vi "Hi_Tec_Control.vi"(0 "Carrier 1 Voltage":dbl(knob) min=0.0 max=5.0 scale=0.0..5.0 scale format="%.1f", 1 "Carrier 2 Voltage":dbl(knob) min=0.0 max=5.0 scale=0.0..5.0 scale format="%.1f", 2 "Trace Voltage":dbl(knob) min=0.0 max=5.0 scale=0.0..5.0 scale format="%.1f", 3 "Trace_2 Voltage":dbl(knob) min=0.0 max=5.0 scale=0.0..5.0 scale format="%.1f", 4 "Client Name":string) -> (5 "Scan Comments":string)   [LabVIEW 2015]
uses:
  ADAM Client/Sub VIs/Channel_State_Control.ctl
  Anemometry/Anemometry Sub Vis/Controls/In_Range.ctl
  ADAM Client/Sub VIs/ADAM Controls/Update_scan_value.ctl
panel:
  out "Second stage":dbl[][](graph)
  out "First stage":dbl[][](graph)
  out "Increasing trace":bool
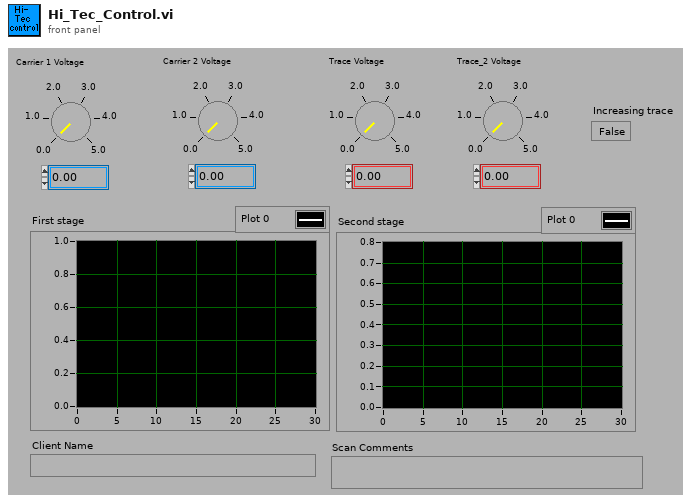
[diagram p1: front panel]
types:
  T1 = typedef "Channel_State_Control.ctl" = enum16{"Channel Name", "Channel Name Starts with", "Main Address"}
  T2 = typedef "In_Range.ctl" = enum16{"%", "±", "% & ±"}
  T3 = typedef "Update_scan_value.ctl" = cluster{"Channel Name":string, "New Value":dbl}
  T4 = enum16{"Append to Global", "Read Global then Clear"}
  T5 = typedef "Ch_description_ADAM.ctl" = cluster{"Ch Name":string, "Type":T6, "Function":T7, "Ch State":T8, "Calibration type":T9, "A":dbl, "B":dbl, "C":dbl, "D":dbl, "Comments":string, "Address":T10, "String":string, "Duty":u16}
  T6 = typedef "Module_type_ADAM.ctl" = string
  T7 = typedef "Function_ADAM.ctl" = enum16{"Analogue Input", "Digital Input", "Event counter", "Event rate", "Analogue Output", "Digital Output", "Relay Output"}
  T8 = typedef "Channel_State.ctl" = enum16{"On", "Off", "Always On", "Always Off"}
  T9 = typedef "Calib_type_ADAM.ctl" = enum16{"Raw", "Bx + A", "Cx^2 + Bx + A", "Dx^3 + Cx^2 + Bx + A", "In Band", "Hi-Tec Q", "Hi-Tec M_dot", "Text"}
  T10 = typedef "Address.ctl" = cluster{"Main":i32, "Ch.":i32, "Sub":i32, "Port Name":string}
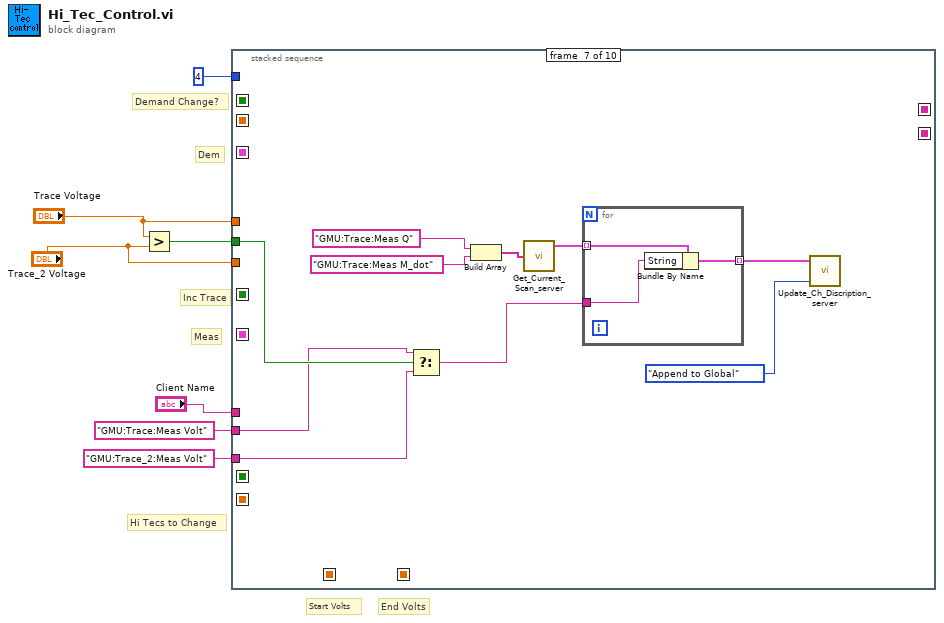
[diagram p0: block diagram]
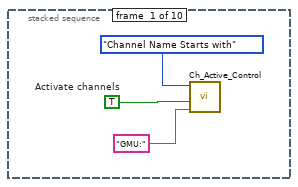
[diagram p2: hidden frame]
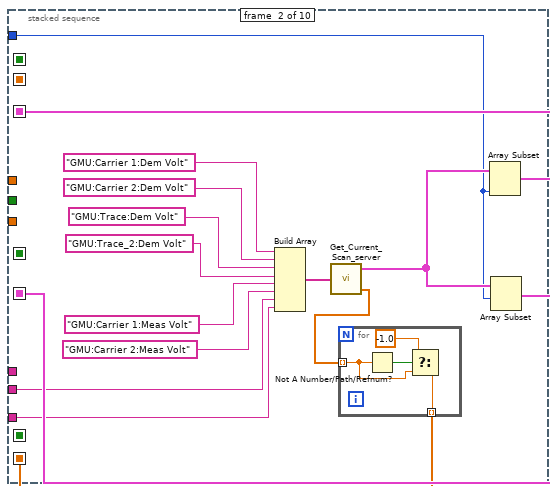
[diagram p3: hidden frame]
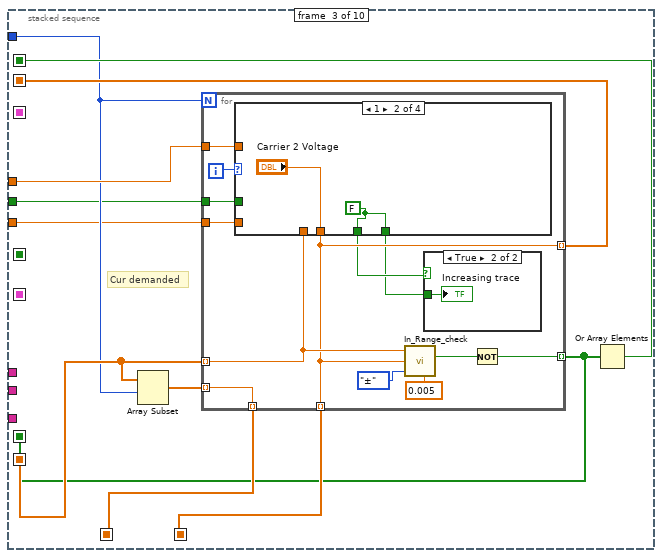
[diagram p4: hidden frame]
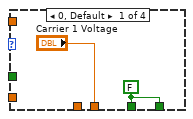
[diagram p6: hidden frame]
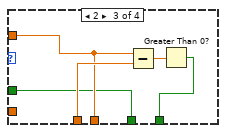
[diagram p7: hidden frame]
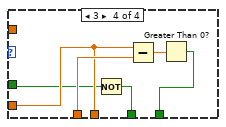
[diagram p8: hidden frame]
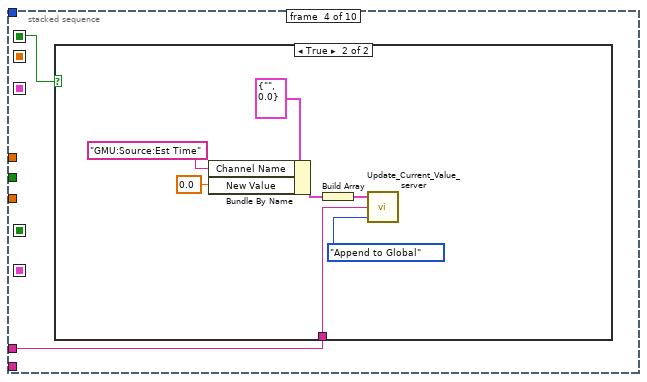
[diagram p9: hidden frame]
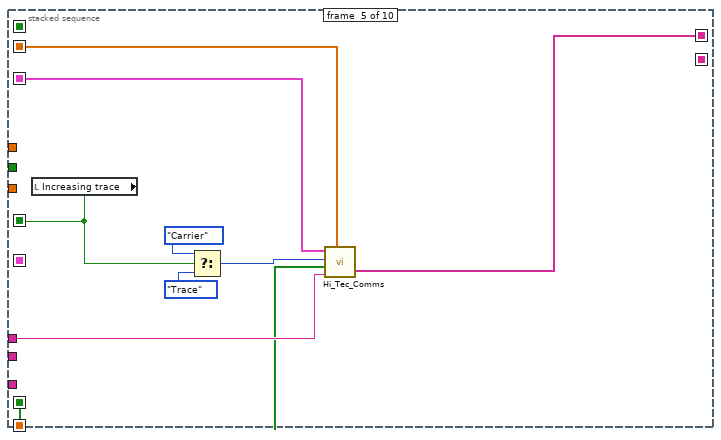
[diagram p11: hidden frame]
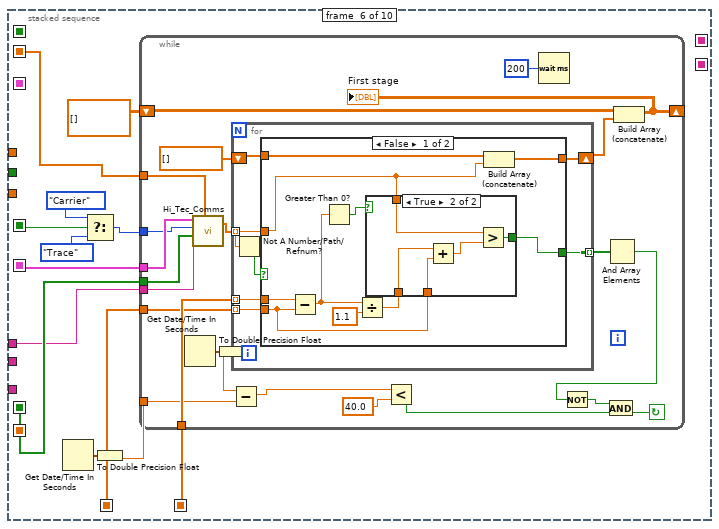
[diagram p12: hidden frame]
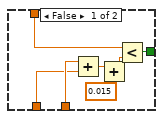
[diagram p13: hidden frame]
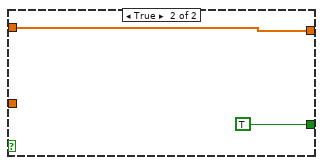
[diagram p14: hidden frame]
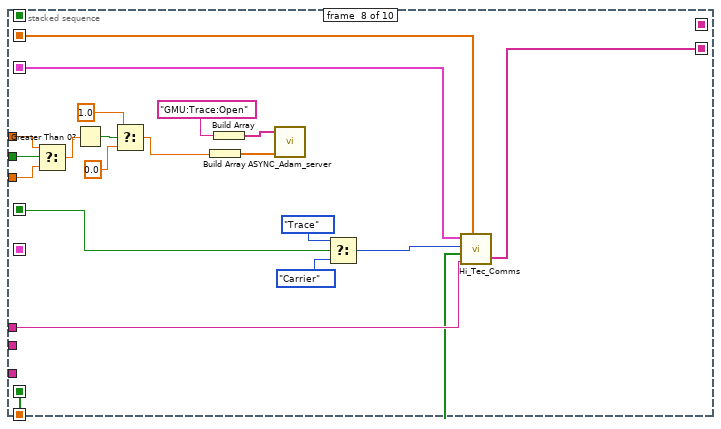
[diagram p15: hidden frame]
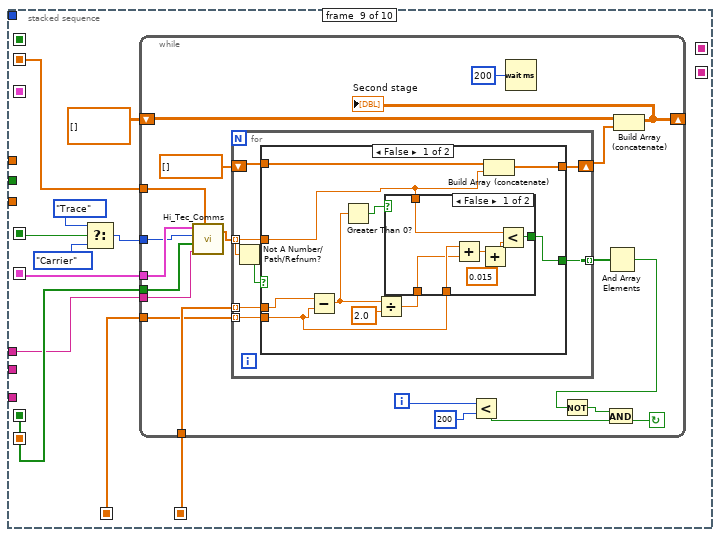
[diagram p16: hidden frame]
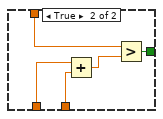
[diagram p17: hidden frame]
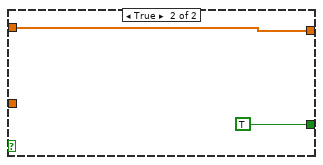
[diagram p18: hidden frame]
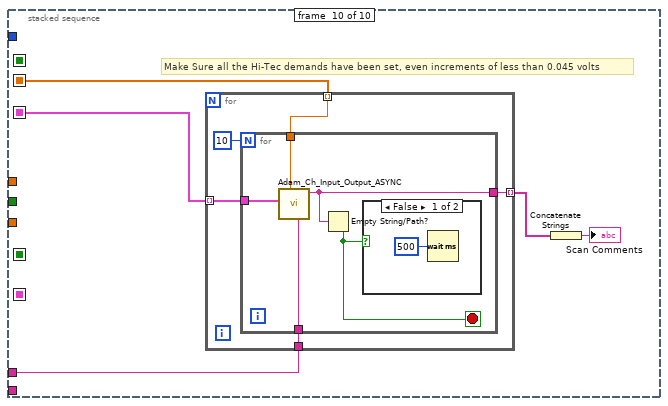
[diagram p19: hidden frame]
diagram:
  # "Dem"
  # "Demand Change?"
  # "End Volts"
  # "Start Volts"
  # "Inc Trace"
  # "Meas"
  # "Hi Tecs to Change"
  n1 = Greater?(x="Trace Voltage", y="Trace_2 Voltage") -> (0:w4:bool)
  n2 = stacked-sequence {
    seq-local: [_ w21 _ _ _ _ _ _ _ _] -> [_ _ _ _ w81 _ _ w174 _ w253]
    seq-local: [_ w16 _ _ _ _ _ _ _ _] -> [_ _ w38 _ _ _ _ _ _ _]
    seq-local: [_ _ w36 _ _ _ _ _ _ _] -> [_ _ _ _ w80 w100 _ w173 w198 _]
    seq-local: [_ w20 _ _ _ _ _ _ _ _] -> [_ _ _ _ _ w96 _ _ w194 _]
    seq-local: [_ _ _ _ w87 _ _ _ _ _] -> [_ _ _ _ _ w97 _ w187 w195 _]
    seq-local: [_ _ w40 _ _ _ _ _ _ _] -> [_ _ _ _ _ w93 _ _ w191 _]
    seq-local: [_ _ w39 _ _ _ _ _ _ _] -> [_ _ _ _ _ w94 _ _ w192 _]
    seq-local: [_ _ w35 _ _ _ _ _ _ _] -> [_ _ _ w70 _ _ _ _ _ _]
    seq-local: [_ _ w33 _ _ _ _ _ _ _] -> [_ _ _ _ w82 w88 _ w175 w188 w252]
    seq-local: [_ _ _ _ w79 _ _ _ _ _] -> [_ _ _ _ _ _ _ _ _ _]
    seq-local: [_ _ _ _ _ _ _ w172 _ _] -> [_ _ _ _ _ _ _ _ _ _]
    tunnel: "Client Name" -> [_ _ _ w71 w83 w90 _ w183 w189 w254]
    tunnel: "Trace Voltage" -> [_ _ w34 _ _ _ _ w170 _ _]
    tunnel: 4 ("Array Length") -> [_ w13 w32 _ _ _ _ _ _ _]
    tunnel: w4 -> [_ _ w31 _ _ _ w160 w171 _ _]
    tunnel: "Trace_2 Voltage" -> [_ _ w30 _ _ _ _ w168 _ _]
    tunnel: "GMU:Trace:Meas Volt" -> [_ w12 _ _ _ _ w159 _ _ _]
    tunnel: "GMU:Trace_2:Meas Volt" -> [_ w11 _ _ _ _ w158 _ _ _]
    frame #0 {
      w8 = TRUE  # Activate channels
      n3 = call "Ch_Active_Control.vi"("Match"="GMU:", "Activate Channels?"=w8, "Control on"=Channel_State_Control."Channel Name Starts with") -> ()  [unwired: 1 in, 2 out]
    }
    frame #1 {
      n4 = Build Array("GMU:Carrier 1:Dem Volt", "GMU:Carrier 2:Dem Volt", "GMU:Trace:Dem Volt", "GMU:Trace_2:Dem Volt", "GMU:Carrier 1:Meas Volt", "GMU:Carrier 2:Meas Volt", w12, w11) -> (w25:string[])
      n5 = call "Get_Current_Scan_server.vi"("Desired Channels"=w25) -> ("Ch Description Array"=w19:T5[], "Numerical Values"=w17:dbl[])  [unwired: 1 out]
      n6 = for {
        tunnel: w17 -> [w28] mode=indexing
        tunnel: [w27] -> w16 mode=indexing
        n7 = Not A Number/Path/Refnum?(number/path/refnum=w28) -> (NaN/Path/Refnum?=w29:bool)
        n8 = Select(t=-1.0, s=w29, f=w28) -> (s? t:f=w27:dbl)
      }
      n9 = Array Subset(array=w19, length=w13) -> (w21:T5[])  [unwired: 1 in]
      n10 = Array Subset(array=w19, index=w13) -> (w20:T5[])  [unwired: 1 in]
    }
    frame #2 {
      # "Cur demanded"
      n11 = Array Subset(array=w38, index=w32) -> (w37:dbl[])  [unwired: 1 in]
      n12 = for {
        N: w32 -> [_]
        tunnel: w38 -> [w48] mode=indexing
        tunnel: [w51] -> w40 mode=indexing
        tunnel: [w45] -> w39 mode=indexing
        tunnel: [w52] -> w36 mode=indexing
        tunnel: w37 -> [w51] mode=indexing
        tunnel: w34 -> [w46]
        tunnel: [w45] -> w33 mode=indexing
        tunnel: w31 -> [w43]
        tunnel: w30 -> [w41]
        i -> [w53]
        n13 = case shown="1" w53 {
          tunnel: ["Carrier 1 Voltage" "Carrier 2 Voltage" w61 w66] -> w45
          tunnel: w48 -> [_ _ w63 w69]
          tunnel: w46 -> [_ _ w61 _]
          tunnel: [w55 w57 w60 w64] -> w44
          tunnel: w43 -> [_ _ w60 w65]
          tunnel: [w55 w57 w59 w67] -> w42
          tunnel: w41 -> [_ _ _ w66]
          frame 0, Default {
            w55 = FALSE
          }
          frame 1 {
            w57 = FALSE
          }
          frame 2 {
            n14 = Subtract(x=w61, y=w63) -> (x-y=w62:dbl)
            n15 = Greater Than 0?(x=w62) -> (x > 0?=w59:bool)
          }
          frame 3 {
            n16 = Not(x=w65) -> (.not. x?=w64:bool)
            n17 = Subtract(x=w66, y=w69) -> (x-y=w68:dbl)
            n18 = Greater Than 0?(x=w68) -> (x > 0?=w67:bool)
          }
        }
        n19 = call "In_Range_check.vi"("±"=0.005 ("%"), "Mode"=In_Range."±", "Value"=w45, "Setpoint"=w48) -> ("In Range"=w47:bool)  [unwired: 1 in, 2 out]
        n20 = case shown="True" w44 {
          tunnel: w42 -> [_ w54]
          frame False {
          }
          frame True {
            "Increasing trace" <- w54
          }
        }
        n21 = Not(x=w47) -> (.not. x?=w52:bool)
      }
      n22 = Or Array Elements(Boolean array=w36) -> (logical OR=w35:bool)
    }
    frame #3 {
      n23 = case shown="True" w70 {
        tunnel: w71 -> [_ w78]
        frame False {
        }
        frame True {
          n24 = Bundle By Name(cluster=T3 {"Channel Name"="", "New Value"=0.0} ("Update Scan Value Cluster"), "Channel Name"="GMU:Source:Est Time", "New Value"=0.0 ("Bundle Element")) -> (w73:T3)
          n25 = Build Array(w73) -> (w72:T3[])
          n26 = call "Update_Current_Value_server.vi"("Mode"=T4."Append to Global", "Client HD name"=w78, "Update array in"=w72) -> ()  [unwired: 1 out]
        }
      }
    }
    frame #4 {
      n27 = local read "Increasing trace"() -> (w87:bool)
      n28 = Select(t=enum16{"Carrier", "Trace"}."Carrier" ("Type"), s=w87, f=enum16{"Carrier", "Trace"}."Trace" ("Type")) -> (s? t:f=w84:enum16{"Carrier", "Trace"})
      n29 = call "Hi_Tec_Comms.vi"("Ch Description Array"=w81, "Type"=w84, "Hi Tec's To Change"=w80, "Client Name"=w83, "Dem Volts"=w82) -> ("Scan comments"=w79:string[])  [unwired: 1 out]
    }
    frame #5 {
      n30 = Get Date/Time In Seconds() -> (seconds since 1Jan1904=w89:timestamp)
      n31 = Select(t=enum16{"Carrier", "Trace"}."Carrier" ("Type"), s=w97, f=enum16{"Carrier", "Trace"}."Trace" ("Type")) -> (s? t:f=w95:enum16{"Carrier", "Trace"})
      n32 = To Double Precision Float(number=w89) -> (double precision float=w91:dbl)
      n33 = while {
        tunnel: w90 -> [w104]
        tunnel: w91 -> [w107]
        shift-left: dbl[][] [] -> [w113]
        shift-right: [w112] -> _
        tunnel: w93 -> [w120]
        tunnel: w94 -> [w121]
        tunnel: w95 -> [w122]
        tunnel: w96 -> [w123]
        tunnel: w100 -> [w114]
        tunnel: w88 -> [w101]
        stop <- w109 continue-if-true
        n34 = Get Date/Time In Seconds() -> (seconds since 1Jan1904=w103:timestamp)
        n35 = call "Hi_Tec_Comms.vi"("Ch Description Array"=w123, "Type"=w122, "Hi Tec's To Change"=w114, "Client Name"=w104, "Dem Volts"=w101) -> ("Outputs"=w119:dbl[])  [unwired: 1 out]
        n36 = To Double Precision Float(number=w103) -> (double precision float=w108:dbl)
        n37 = Subtract(x=w108, y=w107) -> (x-y=w106:dbl)
        n38 = for {
          tunnel: w121 -> [w130] mode=indexing
          tunnel: w120 -> [w129] mode=indexing
          tunnel: w119 -> [w125] mode=indexing
          tunnel: [w128] -> w118 mode=indexing
          shift-right: [w126] -> w115
          shift-left: dbl[] [] -> [w127]
          n39 = Not A Number/Path/Refnum?(number/path/refnum=w125) -> (NaN/Path/Refnum?=w124:bool)
          n40 = case shown="False" w124 {
            tunnel: w130 -> [w137 _]
            tunnel: w129 -> [w133 _]
            tunnel: w125 -> [w132 _]
            tunnel: [w131 TRUE] -> w128
            tunnel: w127 -> [w136 w153]
            tunnel: [w135 w153] -> w126
            frame False {
              n41 = Subtract(x=w137, y=w133) -> (x-y=w139:dbl)
              n42 = Greater Than 0?(x=w139) -> (x > 0?=w138:bool)
              n43 = Divide(x=w139, y=1.1) -> (x/y=w134:dbl)
              n44 = case shown="True" w138 {
                tunnel: w134 -> [w146 w152]
                tunnel: w133 -> [w147 w151]
                tunnel: w132 -> [w145 w149]
                tunnel: [w144 w148] -> w131
                frame False {
                  n45 = Add(x=w147, y=w146) -> (x+y=w143:dbl)
                  n46 = Add(x=w143, y=0.015 ("x")) -> (x+y=w142:dbl)
                  n47 = Less?(x=w145, y=w142) -> (x < y?=w144:bool)
                }
                frame True {
                  n48 = Add(x=w152, y=w151) -> (x+y=w150:dbl)
                  n49 = Greater?(x=w149, y=w150) -> (0:w148:bool)
                }
              }
              n50 = Build Array (concatenate)(w136, w132) -> (w135:dbl[])
            }
            frame True {
            }
          }
        }
        n51 = Less?(x=w106, y=40.0) -> (x < y?=w111:bool)
        n52 = Wait (ms)(milliseconds to wait=u32 200) -> ()  [unwired: 1 out]
        n53 = And Array Elements(Boolean array=w118) -> (logical AND=w117:bool)
        n54 = Not(x=w117) -> (.not. x?=w110:bool)
        n55 = And(x=w110, y=w111) -> (x .and. y?=w109:bool)
        n56 = Build Array (concatenate)(w113, w115) -> (w112:dbl[][])
        "First stage" <- w112
      }
    }
    frame #6 {
      n57 = Select(t=w159, s=w160, f=w158) -> (s? t:f=w157:string)
      n58 = Build Array("GMU:Trace:Meas Q", "GMU:Trace:Meas M_dot") -> (w162:string[])
      n59 = call "Get_Current_Scan_server.vi"("Desired Channels"=w162) -> ("Ch Description Array"=w161:T5[])  [unwired: 2 out]
      n60 = for {
        tunnel: w161 -> [w167] mode=indexing
        tunnel: w157 -> [w166]
        tunnel: [w165] -> w156 mode=indexing
        n61 = Bundle By Name(cluster=w167, "String"=w166) -> (w165:T5)
      }
      n62 = call "Update_Ch_Discription_server.vi"("Mode"=T4."Append to Global", "Channels to update In"=w156) -> ()  [unwired: 1 in, 1 out]
    }
    frame #7 {
      n63 = Select(t=w170, s=w171, f=w168) -> (s? t:f=w169:dbl)
      n64 = Greater Than 0?(x=w169) -> (x > 0?=w182:bool)
      n65 = Select(t=1.0, s=w182, f=0.0) -> (s? t:f=w179:dbl)
      n66 = Build Array(w179) -> (w176:dbl[])
      n67 = Build Array("GMU:Trace:Open") -> (w177:string[])
      n68 = call "ASYNC_Adam_server.vi"("Values"=w176, "Channel Names"=w177) -> ()  [unwired: 2 in, 2 out]
      n69 = Select(t=enum16{"Carrier", "Trace"}."Trace" ("Type"), s=w187, f=enum16{"Carrier", "Trace"}."Carrier" ("Type")) -> (s? t:f=w184:enum16{"Carrier", "Trace"})
      n70 = call "Hi_Tec_Comms.vi"("Ch Description Array"=w174, "Type"=w184, "Hi Tec's To Change"=w173, "Client Name"=w183, "Dem Volts"=w175) -> ("Scan comments"=w172:string[])  [unwired: 1 out]
    }
    frame #8 {
      n71 = Select(t=enum16{"Carrier", "Trace"}."Trace" ("Type"), s=w195, f=enum16{"Carrier", "Trace"}."Carrier" ("Type")) -> (s? t:f=w193:enum16{"Carrier", "Trace"})
      n72 = while {
        tunnel: w189 -> [w201]
        shift-left: dbl[][] [] -> [w208]
        shift-right: [w202] -> _
        tunnel: w191 -> [w215]
        tunnel: w192 -> [w216]
        tunnel: w193 -> [w217]
        tunnel: w194 -> [w218]
        tunnel: w198 -> [w209]
        tunnel: w188 -> [w199]
        i -> [w204]
        stop <- w203 continue-if-true
        n73 = call "Hi_Tec_Comms.vi"("Ch Description Array"=w218, "Type"=w217, "Hi Tec's To Change"=w209, "Client Name"=w201, "Dem Volts"=w199) -> ("Outputs"=w214:dbl[])  [unwired: 1 out]
        n74 = for {
          tunnel: w216 -> [w225] mode=indexing
          tunnel: w215 -> [w224] mode=indexing
          tunnel: w214 -> [w220] mode=indexing
          tunnel: [w223] -> w213 mode=indexing
          shift-right: [w221] -> w210
          shift-left: dbl[] [] -> [w222]
          n75 = Not A Number/Path/Refnum?(number/path/refnum=w220) -> (NaN/Path/Refnum?=w219:bool)
          n76 = case shown="False" w219 {
            tunnel: w225 -> [w229 _]
            tunnel: w224 -> [w228 _]
            tunnel: w220 -> [w227 _]
            tunnel: [w226 TRUE] -> w223
            tunnel: w222 -> [w235 w248]
            tunnel: [w234 w248] -> w221
            frame False {
              n77 = Subtract(x=w229, y=w228) -> (x-y=w232:dbl)
              n78 = Greater Than 0?(x=w232) -> (x > 0?=w231:bool)
              n79 = Divide(x=w232, y=2.0) -> (x/y=w230:dbl)
              n80 = case shown="False" w231 {
                tunnel: w230 -> [w241 w247]
                tunnel: w228 -> [w242 w246]
                tunnel: w227 -> [w240 w244]
                tunnel: [w239 w243] -> w226
                frame False {
                  n81 = Add(x=w242, y=w241) -> (x+y=w238:dbl)
                  n82 = Add(x=w238, y=0.015 ("x")) -> (x+y=w237:dbl)
                  n83 = Less?(x=w240, y=w237) -> (x < y?=w239:bool)
                }
                frame True {
                  n84 = Add(x=w247, y=w246) -> (x+y=w245:dbl)
                  n85 = Greater?(x=w244, y=w245) -> (0:w243:bool)
                }
              }
              n86 = Build Array (concatenate)(w235, w227) -> (w234:dbl[])
            }
            frame True {
            }
          }
        }
        n87 = Less?(x=w204, y=200) -> (x < y?=w206:bool)
        n88 = Wait (ms)(milliseconds to wait=u32 200) -> ()  [unwired: 1 out]
        n89 = And Array Elements(Boolean array=w213) -> (logical AND=w212:bool)
        n90 = Not(x=w212) -> (.not. x?=w205:bool)
        n91 = And(x=w205, y=w206) -> (x .and. y?=w203:bool)
        n92 = Build Array (concatenate)(w208, w210) -> (w202:dbl[][])
        "Second stage" <- w202
      }
    }
    frame #9 {
      # "Make Sure all the Hi-Tec demands have been set, even increments of less than 0.045 volts"
      n93 = for {
        tunnel: w253 -> [w259] mode=indexing
        tunnel: w254 -> [w257]
        tunnel: w252 -> [w258] mode=indexing
        tunnel: [w256] -> w251 mode=indexing
        n94 = for {
          N: 10 -> [_]
          tunnel: w259 -> [w264]
          tunnel: w258 -> [w263]
          tunnel: w257 -> [w262]
          tunnel: [w261] -> w256
          stop <- w260 stop-if-true
          n95 = call "Adam_Ch_Input_Output_ASYNC.vi"("Client Name"=w262, "Value to Output"=w263, "Ch Discription"=w264) -> ("Scan comment"=w261:string)  [unwired: 4 in, 4 out]
          n96 = Empty String/Path?(string/path=w261) -> (empty?=w260:bool)
          n97 = case shown="False" w260 {
            frame False {
              n98 = Wait (ms)(milliseconds to wait=u32 500) -> ()  [unwired: 1 out]
            }
            frame True {
            }
          }
        }
      }
      n99 = Concatenate Strings(w251) -> (→"Scan Comments":string)
    }
  }
